vi "configure.vi"(8 "error in (no error)":errorcluster, 11 "GenericPlugin in":refnum<class "TrajectoryRK110916Throughput.lvclass">) -> (0 "error out":errorcluster, 3 "GenericPlugin out":refnum<class "TrajectoryRK110916Throughput.lvclass">)   [LabVIEW 2010, in "TrajectoryRK110916Throughput.lvclass"]
doc: "The dynamic dispatch version of this VI loads and displays the configuration file associated with the plug-in object. The user modify and save the configuration data."
uses:
  TrajectoryRK110916Throughput.lvclass
  TrajectoryRK110916Throughput.lvclass/TrajectoryRK110916Throughput.ctl
  common/classes/GenericComponent/GenericComponent/GenericComponent.lvclass
panel:
  in  "cancel":bool
  in  "save":bool
  in  "Tab Control":enum32{"Description", "Settings"}(tab)
  in  "FGPA clockspeed":dbl caption="Hz"
  in  "Data rate":u32 caption="Samples/sec"
  out "configuration name":string
  # "Configure TrajectoryThroughput"
  # "Throughput test"
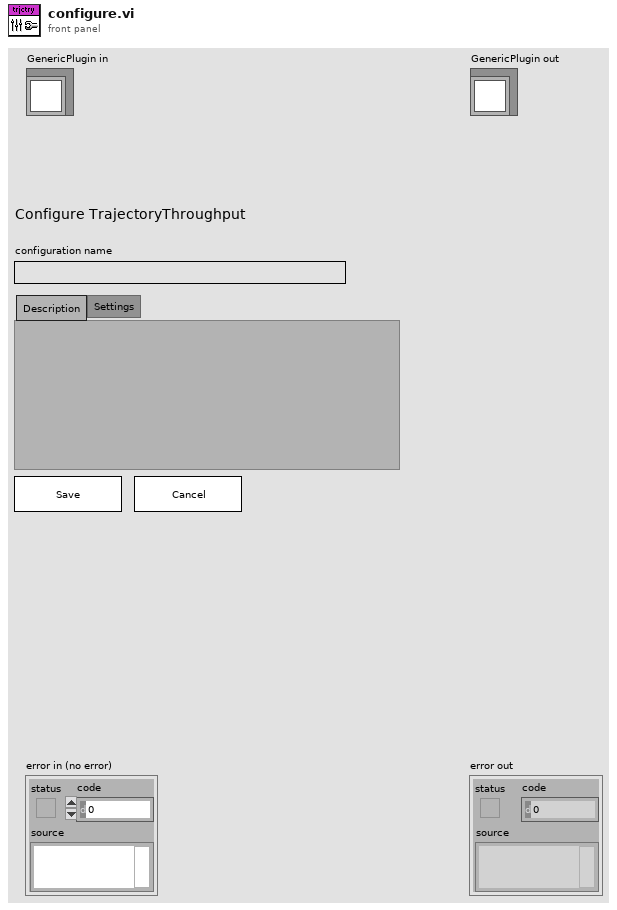
[diagram p1: front panel]
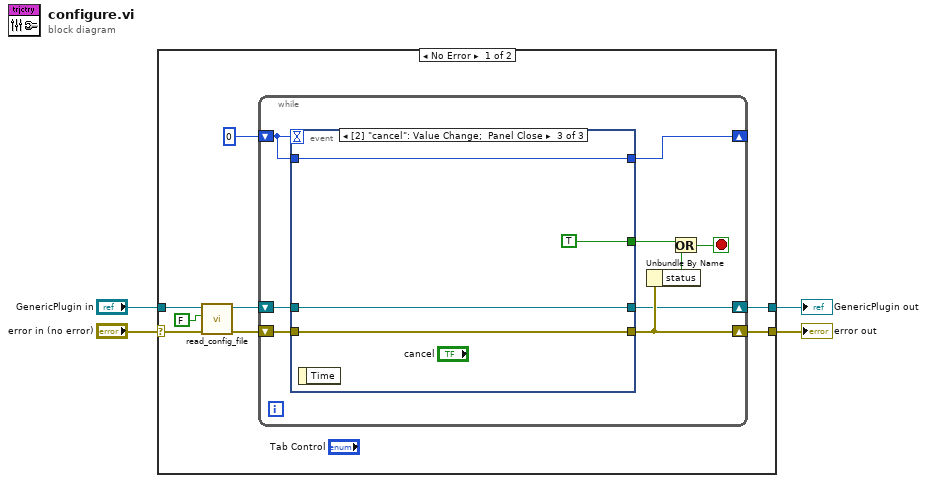
[diagram p0: block diagram]
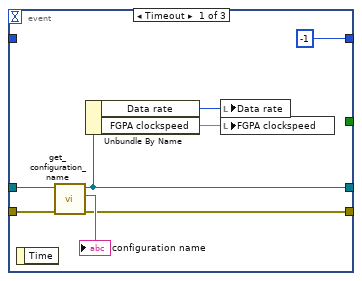
[diagram p2: hidden frame]
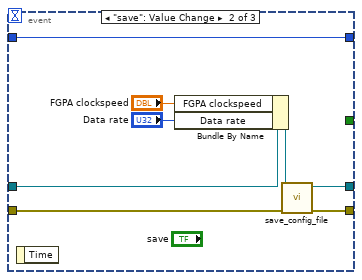
[diagram p3: hidden frame]
diagram:
  n1 = case shown="No Error" "error in (no error)" {
    selector: "error in (no error)" -> [w12 w43]
    tunnel: [w6 w43] -> w3
    tunnel: "GenericPlugin in" -> [w11 w42]
    tunnel: [w5 w42] -> w1
    frame No Error {
      n2 = call-dynamic "read_config_file.vi"("error in (no error)"=w12, "force load?"=FALSE, "GenericPlugin in"=w11) -> ("error out"=w9:errorcluster, "GenericPlugin out"=w7:refnum<class "TrajectoryRK110916Throughput.lvclass">)  [unwired: 7 out]
      n3 = while {
        shift-right: [w17] -> w6
        shift-left: w9 -> [w21]
        shift-right: [w19] -> _
        shift-left: 0 -> [w20]
        shift-right: [w16] -> w5
        shift-left: w7 -> [w18]
        stop <- w13 stop-if-true
        n4 = event shown="[2] \"cancel\": Value Change;  Panel Close" {
          selector: _ -> [_ _ _]
          dyn-events: _ -> [_ _ _]
          timeout: w20 -> [_ _ _]
          tunnel: w21 -> [w29 w36 w41]
          tunnel: w18 -> [w28 w33 w39]
          tunnel: [w26 w35 w41] -> w17
          tunnel: w20 -> [_ w37 w40]
          tunnel: [-1 w37 w40] -> w19
          tunnel: [w22 w34 w39] -> w16
          tunnel: [_ _ TRUE] -> w14
          event Timeout {
            n5 = event-data() -> ()  [unwired: 1 in, 1 out]
            n6 = call "get_configuration_name.vi"("error in (no error)"=w29, "GenericPlugin.lvclass in"=w28) -> ("error out"=w26:errorcluster, "configuration name"=→"configuration name":string, "GenericPlugin.lvclass out"=w22:refnum<class "TrajectoryRK110916Throughput.lvclass">)  [unwired: 7 in]
            n7 = Unbundle By Name(w22) -> ("Data rate"=w25:u32, "FGPA clockspeed"=w24:dbl)
            n8 = local write "Data rate"(w25) -> ()
            n9 = local write "FGPA clockspeed"(w24) -> ()
          }
          event "save": Value Change {
            n10 = event-data() -> ()  [unwired: 1 in, 1 out]
            n11 = Bundle By Name(cluster=w33, "FGPA clockspeed"="FGPA clockspeed", "Data rate"="Data rate") -> (w32:refnum<class "TrajectoryRK110916Throughput.lvclass">)
            n12 = call-dynamic "save_config_file.vi"("error in (no error)"=w36, "GenericPlugin in"=w32) -> ("error out"=w35:errorcluster, "GenericPlugin out"=w34:refnum<class "TrajectoryRK110916Throughput.lvclass">)  [unwired: 2 in, 6 out]
          }
          event "cancel": Value Change; Panel Close {
            n13 = event-data() -> ()  [unwired: 1 in, 1 out]
          }
        }
        n14 = Unbundle By Name(w17) -> ("status"=w15:bool)
        n15 = Or(x=w14, y=w15) -> (x .or. y?=w13:bool)
      }
    }
    frame Error {
    }
  }
  "error out" <- w3
  "GenericPlugin out" <- w1
